vi "Read Server Controller Enqueuer.vi"(8 "error in (no error)":errorcluster, 11 "WS Server in":refnum<class "WS Server.lvclass">) -> (0 "error out":errorcluster, 2 "Actor Framework:Message Enqueuer":refnum<class "Message Enqueuer.lvclass">, 3 "WS Server out":refnum<class "WS Server.lvclass">)   [LabVIEW 2016, in "WebSocket Networking.lvlib" / "WS Server.lvclass"]
uses:
  <userlib>/Common Components/WebSocket Networking/WS Server/WS Server.lvclass
  <vilib>/ActorFramework/Message Enqueuer/Message Enqueuer.lvclass
  <userlib>/Common Components/WebSocket Networking/WS Server/WS Server.lvclass/WS Server.ctl
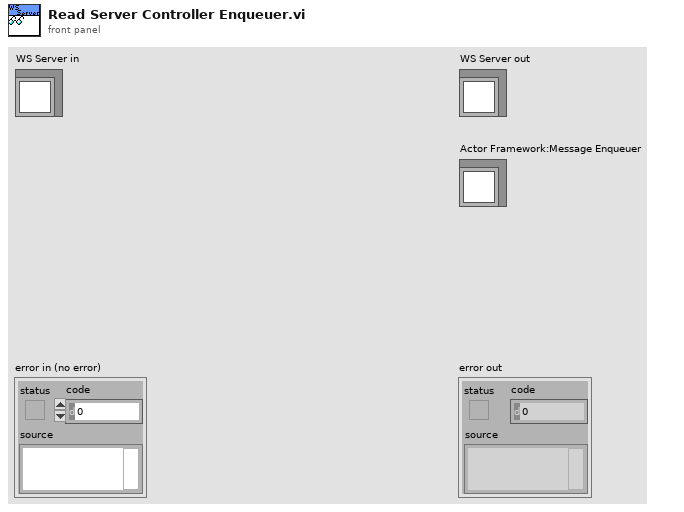
[diagram p1: front panel]
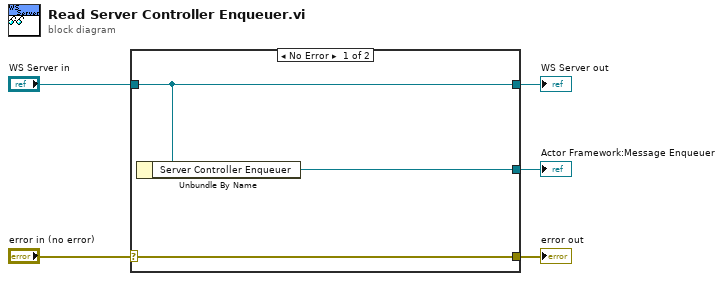
[diagram p0: block diagram]
diagram:
  n1 = case shown="No Error" "error in (no error)" {
    selector: "error in (no error)" -> [w8 w9]
    tunnel: [w8 w9] -> w4
    tunnel: [w7 w10] -> w2
    tunnel: "WS Server in" -> [w7 w10]
    tunnel: [w6 _] -> w1
    frame No Error {
      n2 = Unbundle By Name(w7) -> ("Server Controller Enqueuer"=w6:refnum<class "Message Enqueuer.lvclass">)
    }
    frame Error {
    }
  }
  "error out" <- w4
  "WS Server out" <- w2
  "Actor Framework:Message Enqueuer" <- w1
